vi "5024_set_output.vi"(0 "Set to:":dbl min=0.0 max=20.0 format="%.3f", 1 "Address (all reqd.)":T1, 2 "Channel Name":string) -> (3 "Comment":string, 6 "Good Reply":bool)   [LabVIEW 2018]
uses:
  ADAM Client/Sub VIs/ADAM Controls/Address.ctl
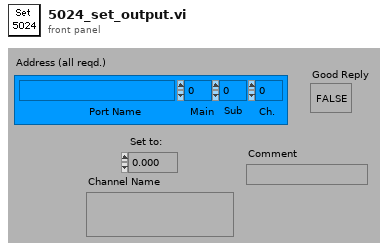
[diagram p1: front panel]
types:
  T1 = typedef "Address.ctl" = cluster{"Main":i32, "Ch.":i32, "Sub":i32, "Port Name":string}
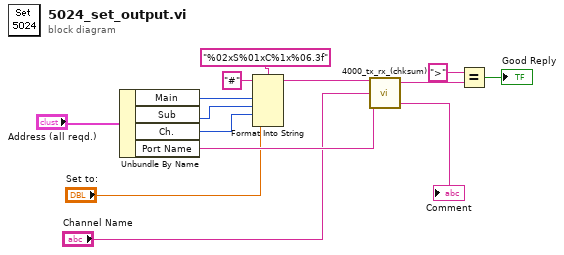
[diagram p0: block diagram]
diagram:
  n1 = Unbundle By Name("Address (all reqd.)") -> ("Main"=w13:i32, "Sub"=w14:i32, "Ch."=w7:i32, "Port Name"=w6:string)
  n2 = Format Into String(format string="%02xS%01xC%1x%06.3f", initial string="#", w13, w14, w7, "Set to:") -> (resulting string=w10:string)  [unwired: 1 in, 1 out]
  n3 = call "4000_tx_rx_(chksum).vi"("Write String"=w10, "Channel Name"="Channel Name", "Port Name"=w6) -> ("Read"=w4:string, "Comment out"=→"Comment":string)  [unwired: 2 in, 1 out]
  n4 = Equal?(x=">", y=w4) -> (x = y?=→"Good Reply":bool)
